vi "Draw Project Results Table Constants.vi"(8 "error in":errorcluster, 9 "Constant Results":string[][](array[string]), 11 "Project Results Ref":refnum<vi>) -> (0 "error out":errorcluster)   [LabVIEW 2020, in "ConstantErrorsMaker.lvlib"]
uses:
  ConstantErrorsMaker.lvlib
  <vilib>/Utility/miscctls.llb/LVRowAndColumnTypeDef.ctl
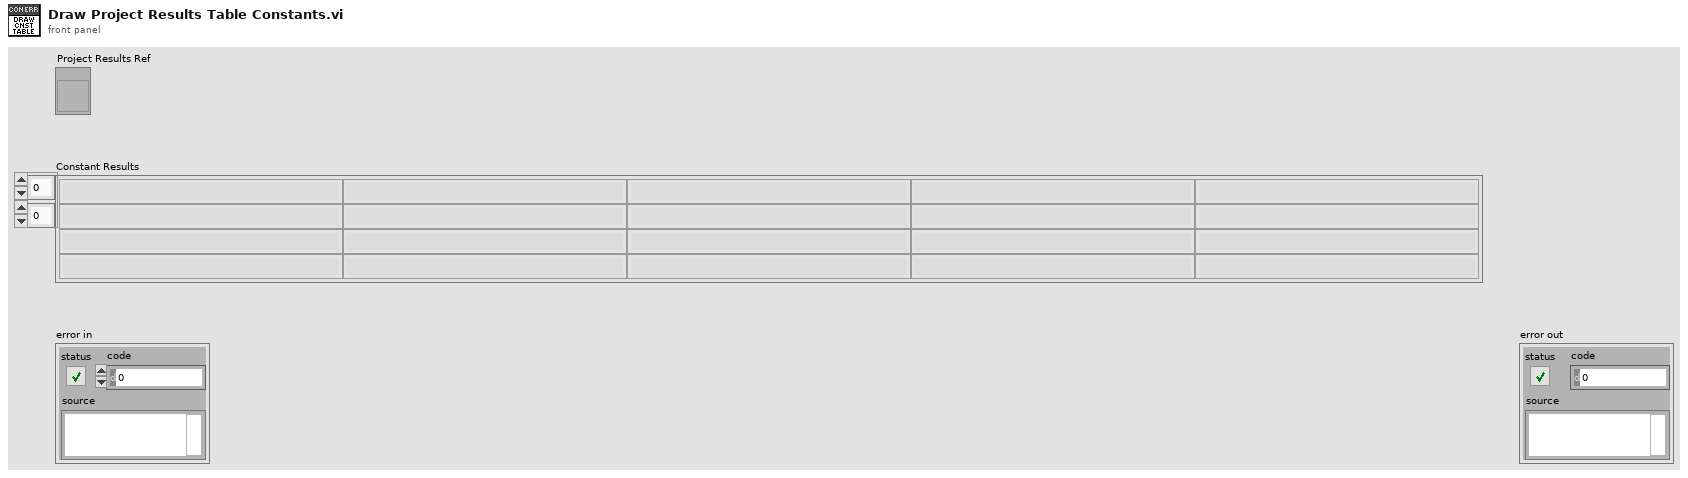
[diagram p1: front panel]
types:
  T1 = typedef "LVRowAndColumnTypeDef.ctl" = cluster{"Row":i32, "Column":i32}
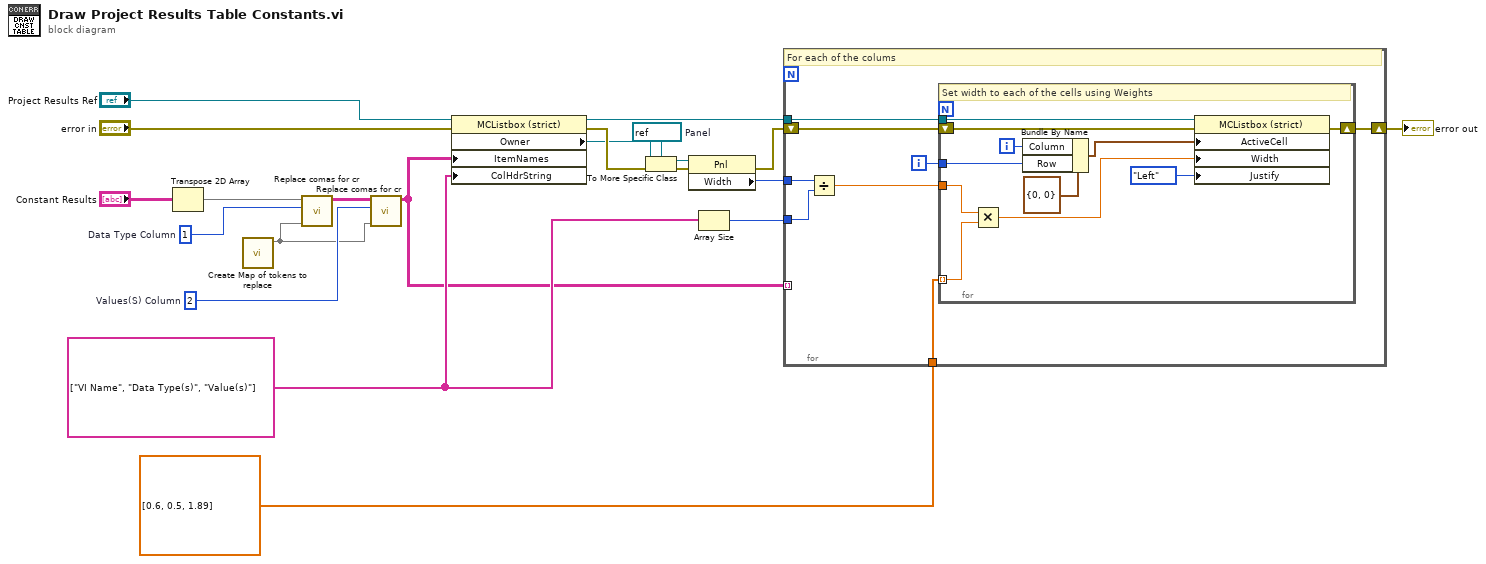
[diagram p0: block diagram]
diagram:
  w4 = 2  # Values(S) Column
  w6 = 1  # Data Type Column
  w9 = string[] ["VI Name", "Data Type(s)", "Value(s)"] ("Column Header Strings[] 2")
  w14 = refnum<vi> refnum  # Panel
  n1 = Transpose 2D Array(2D array="Constant Results") -> (transposed array=w2:string[][])
  n2 = call "Create Map of tokens to replace.vi"() -> ("Tokens to replace"=w1:map{string, string})  [unwired: 11 in]
  n3 = call "Replace comas for cr.vi"("Tokens to replace"=w1, "Col to Replace CR"=w6, "Array in"=w2) -> ("Array Replaced"=w5:string[][])  [unwired: 8 in]
  n4 = call "Replace comas for cr.vi"("Tokens to replace"=w1, "Col to Replace CR"=w4, "Array in"=w5) -> ("Array Replaced"=w3:string[][])  [unwired: 8 in]
  n5 = property on="Property Node" class="MCListbox (strict)"(reference="Project Results Ref", error in="error in", "ItemNames"=w3, "ColHdrString"=w9) -> (reference out=w13:refnum<vi>, error out=w19:errorcluster, "Owner"=w12:refnum<vi>)
  n6 = To More Specific Class(target class=w14, reference=w12, error in=w19) -> (specific class reference=w15:refnum<vi>, error out=w20:errorcluster)
  n7 = property class="Pnl"(reference=w15, error in=w20) -> (error out=w21:errorcluster, "Width"=w16:u32)  [unwired: 1 out]
  n8 = Array Size(array=w9) -> (size(s)=w10:i32)
  n9 = for {
    tunnel: w16 -> [w26]
    tunnel: w13 -> [w25]
    shift-right: [w28] -> w17
    shift-left: w21 -> [w29]
    tunnel: w3 -> [_] mode=indexing
    tunnel: w10 -> [w23]
    tunnel: dbl[] [0.6, 0.5, 1.89] ("Weights") -> [w22]
    i -> [w24]
    # "For each of the colums"
    n10 = Divide(x=w26, y=w23) -> (x/y=w27:dbl)
    n11 = for {
      tunnel: w27 -> [w36]
      tunnel: w22 -> [w34] mode=indexing
      tunnel: w25 -> [w33]
      shift-right: [w39] -> w28
      shift-left: w29 -> [w40]
      tunnel: w24 -> [w32]
      i -> [w37]
      # "Set width to each of the cells using Weights"
      n12 = Multiply(x=w36, y=w34) -> (x*y=w35:dbl)
      n13 = Bundle By Name(cluster=T1 {"Row"=0, "Column"=0} ("Active Cell:Active Cell"), "Column"=w37, "Row"=w32) -> (w38:T1)
      n14 = property class="MCListbox (strict)"(reference=w33, error in=w40, "ActiveCell"=w38, "Width"=w35, "Justify"=enum16{"Left", "Center", "Right"}."Left" ("Active Cell:Cell Justification")) -> (error out=w39:errorcluster)  [unwired: 1 out]
    }
  }
  "error out" <- w17
